vi "multiply.vi"(8 "error in (no error)":errorcluster, 10 "factor":dbl, 11 "ImageCollection in":refnum<class "ImageCollection.lvclass">) -> (0 "error out":errorcluster, 3 "ImageCollection out":refnum<class "ImageCollection.lvclass">)   [LabVIEW 2010, in "ImageCollection.lvclass"]
uses:
  ImageCollection.lvclass
  Image/Image/Image.lvclass
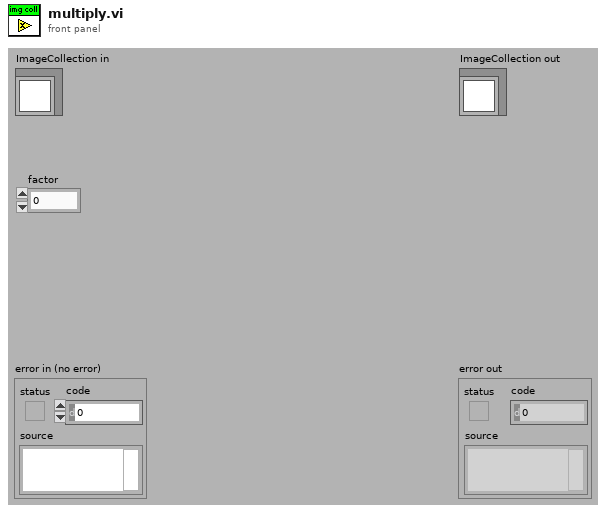
[diagram p1: front panel]
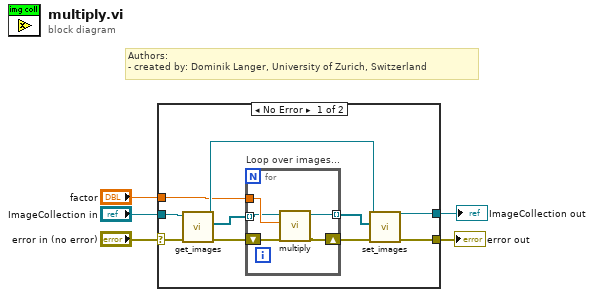
[diagram p0: block diagram]
diagram:
  # "Authors: \n- created by: Dominik Langer, University of Zurich, Switzerland"
  n1 = case shown="No Error" "error in (no error)" {
    selector: "error in (no error)" -> [w15 w22]
    tunnel: [w12 w22] -> w4
    tunnel: [w9 w21] -> w2
    tunnel: "ImageCollection in" -> [w11 w21]
    tunnel: "factor" -> [w8 _]
    frame No Error {
      n2 = call-dynamic "get_images.vi"("error in (no error)"=w15, "ImageCollection.lvclass in"=w11) -> ("error out"=w14:errorcluster, "images"=w7:refnum<class "Image.lvclass">[], "ImageCollection.lvclass out"=w10:refnum<class "ImageCollection.lvclass">)  [unwired: 7 out]
      n3 = for "Loop over images..." {
        shift-right: [w16] -> w13
        shift-left: w14 -> [w20]
        tunnel: w8 -> [w19]
        tunnel: w7 -> [w18] mode=indexing
        tunnel: [w17] -> w6 mode=indexing
        n4 = call-dynamic "multiply.vi"("error in (no error)"=w20, "factor"=w19, "Image in"=w18) -> ("error out"=w16:errorcluster, "Image out"=w17:refnum<class "Image.lvclass">)  [unwired: 1 in, 6 out]
      }
      n5 = call-dynamic "set_images.vi"("error in (no error)"=w13, "images"=w6, "ImageCollection.lvclass in"=w10) -> ("error out"=w12:errorcluster, "ImageCollection.lvclass out"=w9:refnum<class "ImageCollection.lvclass">)  [unwired: 7 out]
    }
    frame Error {
    }
  }
  "error out" <- w4
  "ImageCollection out" <- w2
